vi "BDF-Read Records.vi"(0 "Path":path, 5 "Header":T1, 7 "First record":i32, 9 "Num records":i32=1, 11 "error in (no error)":errorcluster) -> (8 "Data (uV)":dbl[][](array[numeric]), 10 "status array":u8[][](array[numeric]), 15 "error out":errorcluster)   [LabVIEW 2015]
uses:
  BDF-Header.ctl
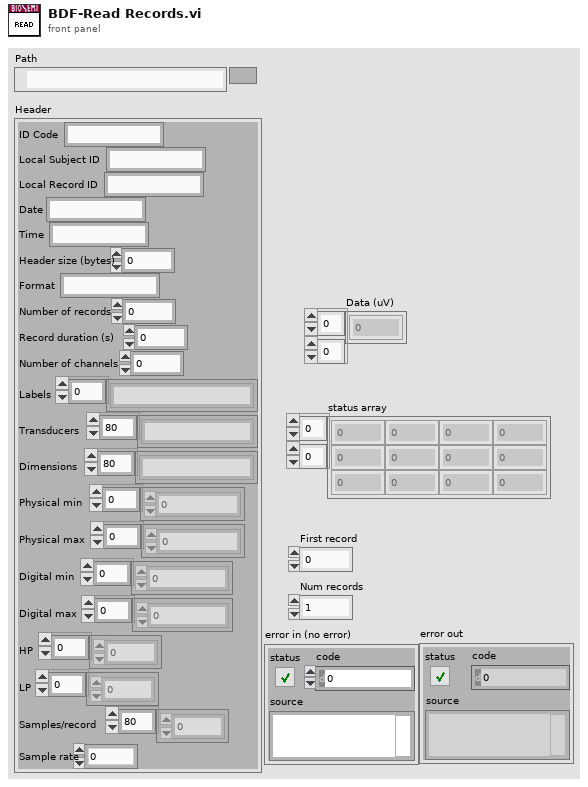
[diagram p1: front panel]
types:
  T1 = typedef "BDF-Header.ctl" = cluster{"ID Code":string, "Local Subject ID":string, "Local Record ID":string, "Date":string, "Time":string, "Header size (bytes)":i32, "Format":string, "Number of records":i32, "Record duration (s)":dbl, "Number of channels":i32, "Labels":string[], "Transducers":string[], "Dimensions":string[], "Physical min":dbl[], "Physical max":dbl[], "Digital min":i32[], "Digital max":i32[], "HP":dbl[], "LP":dbl[], "Samples/record":i32[], "Sample rate":dbl}
  T2 = enum16{"open", "replace", "create", "open or create", "replace or create", "replace or create with confirmation"}
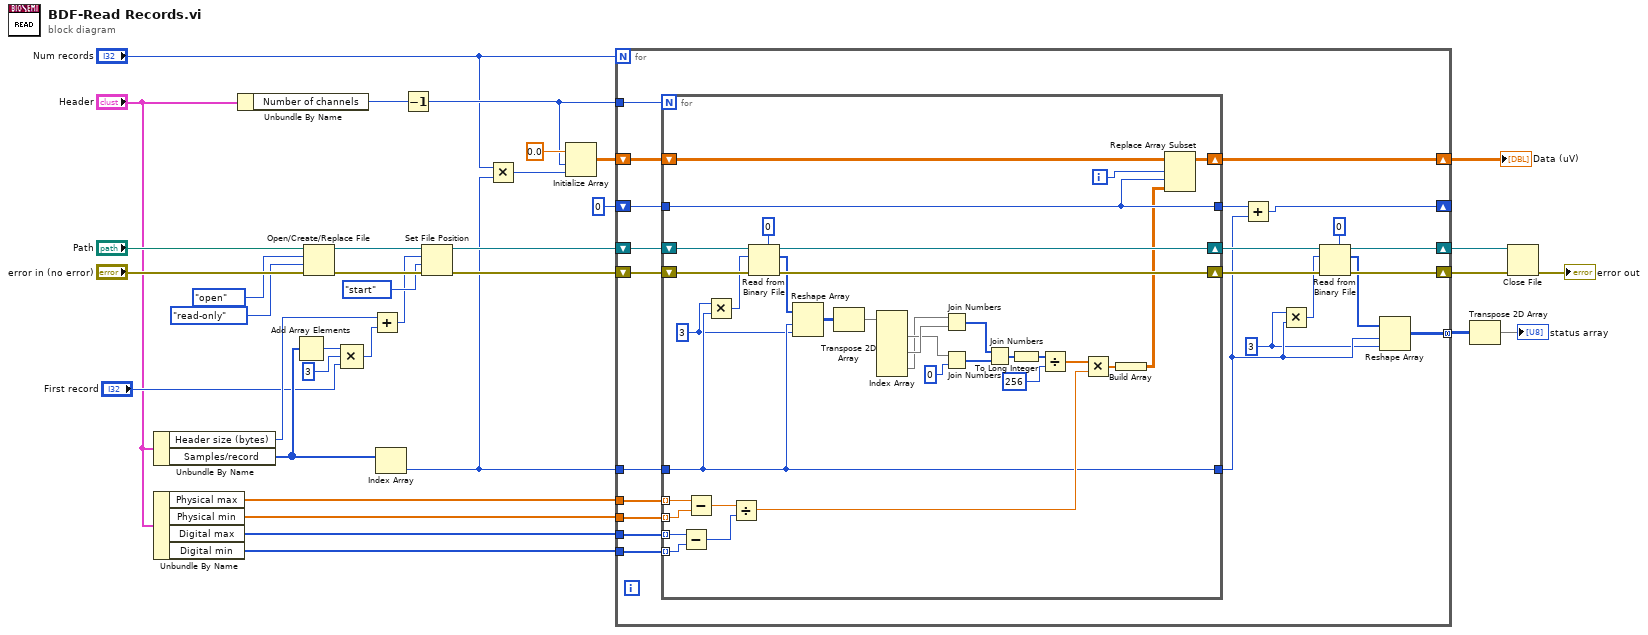
[diagram p0: block diagram]
diagram:
  n1 = Unbundle By Name("Header") -> ("Header size (bytes)"=w17:i32, "Samples/record"=w19:i32[])
  n2 = Unbundle By Name("Header") -> ("Physical max"=w23:dbl[], "Physical min"=w22:dbl[], "Digital max"=w21:i32[], "Digital min"=w20:i32[])
  n3 = Unbundle By Name("Header") -> ("Number of channels"=w13:i32)
  n4 = Add Array Elements(numeric array=w19) -> (sum=w18:i32)
  n5 = Open/Create/Replace File(file path (use dialog)="Path", error in="error in (no error)", operation (0:open)=T2."open", access (0:read/write)=enum16{"read/write", "read-only", "write-only"}."read-only") -> (refnum out=w30:refnum<file>, error out=w31:errorcluster)  [unwired: 2 in, 1 out]
  n6 = Compound Arithmetic op=MULTIPLY(w18, 3, "First record") -> (w15:i32)
  n7 = Add(x=w17, y=w15) -> (x+y=w14:i32)
  n8 = Index Array(array=w19) -> (element=w2:i32)  [unwired: 1 in]
  n9 = Decrement(x=w13) -> (x-1=w10:i32)
  n10 = Set File Position(offset (in bytes) (0)=w14, refnum=w30, from (0:start)=enum16{"start", "end", "current"}."start", error in=w31) -> (refnum out=w27:refnum<file>, error out=w28:errorcluster)
  n11 = Multiply(x="Num records", y=w2) -> (x*y=w8:i32)
  n12 = Initialize Array(0.0 ("element"), w10, w8) -> (w7:dbl[][])
  n13 = for {
    N: "Num records" -> [_]
    tunnel: w2 -> [w58]
    shift-right: [w43] -> w25
    shift-left: w28 -> [w57]
    shift-right: [w36] -> w26
    shift-left: w27 -> [w56]
    tunnel: w23 -> [w55]
    tunnel: w22 -> [w54]
    tunnel: w21 -> [w53]
    tunnel: w20 -> [w52]
    tunnel: w10 -> [w51]
    shift-right: [w49] -> w6
    shift-left: w7 -> [w50]
    shift-right: [w46] -> _
    shift-left: 0 -> [w48]
    tunnel: [w40] -> w4 mode=concatenating
    w38 = 3
    n14 = for {
      N: w51 -> [_]
      tunnel: w58 -> [w70]
      shift-right: [w87] -> w45
      shift-left: w56 -> [w92]
      shift-right: [w90] -> w44
      shift-left: w57 -> [w91]
      tunnel: w55 -> [w86] mode=indexing
      tunnel: w54 -> [w85] mode=indexing
      tunnel: w53 -> [w84] mode=indexing
      tunnel: w52 -> [w83] mode=indexing
      shift-right: [w79] -> w49
      shift-left: w50 -> [w78]
      tunnel: w48 -> [w77]
      tunnel: [w77] -> w47
      tunnel: [w70] -> w39
      i -> [w68]
      w69 = 3
      n15 = Subtract(x=w84, y=w83) -> (x-y=w81:i32)
      n16 = Subtract(x=w86, y=w85) -> (x-y=w82:dbl)
      n17 = Multiply(x=w69, y=w70) -> (x*y=w88:i32)
      n18 = Divide(x=w82, y=w81) -> (x/y=w80:dbl)
      n19 = Read from Binary File(5:u8 0 ("Numeric"), 8:w91, 10:w88, 11:w92) -> (0:w90:errorcluster, 2:w76:u8[], 3:w87:refnum<file>)  [unwired: 2 in, 1 out]
      n20 = Reshape Array(w76, w70, w69) -> (w59:u8[][])
      n21 = Transpose 2D Array(2D array=w59) -> (transposed array=w60:u8[][])
      n22 = Index Array(array=w60) -> (element #1=w71:u8[], element #2=w72:u8[], element #3=w67:u8[])  [unwired: 6 in]
      n23 = Join Numbers(hi=w67, lo=w72) -> ((hi.lo)=w75:u16[])
      n24 = Join Numbers(hi=w71, lo=u8 0) -> ((hi.lo)=w74:u16[])
      n25 = Join Numbers(hi=w75, lo=w74) -> ((hi.lo)=w66:u32[])
      n26 = To Long Integer(number=w66) -> (32bit integer=w65:i32[])
      n27 = Divide(x=w65, y=256) -> (x/y=w61:dbl[])
      n28 = Multiply(x=w61, y=w80) -> (x*y=w62:dbl[])
      n29 = Build Array(w62) -> (w63:dbl[][])
      n30 = Replace Array Subset(array=w78, new element=w63, index (row)=w68, index (col)=w77) -> (w79:dbl[][])
    }
    n31 = Add(x=w47, y=w39) -> (x+y=w46:i32)
    n32 = Multiply(x=w38, y=w39) -> (x*y=w42:i32)
    n33 = Read from Binary File(5:u8 0 ("Numeric"), 8:w44, 10:w42, 11:w45) -> (0:w43:errorcluster, 2:w41:u8[], 3:w36:refnum<file>)  [unwired: 2 in, 1 out]
    n34 = Reshape Array(w41, w39, w38) -> (w40:u8[][])
  }
  "Data (uV)" <- w6
  n35 = Transpose 2D Array(2D array=w4) -> (transposed array=→"status array":u8[][])
  n36 = Close File(refnum=w26, error in=w25) -> (error out=→"error out":errorcluster)  [unwired: 1 out]
